vi "Handle Picture Shortcut Activation.vi"(8 "MenuRef":refnum<k9>, 9 "Container State":T1, 10 "state in":T2={"Draw Options"={"Background Color"=16777215, "Grid Color"=13816530, "Angle Units"=enum."Radians", "Draw Solid Background"=TRUE, "Draw Grid"=TRUE, "Grid Spacing"=1.0, "AutoScale"=TRUE, "Fit to Radius"=1.0, "data row options"=[]}}, 11 "data in":T6) -> ()   [LabVIEW 2017, in "NI_Robotics_2D Rangefinder.xctl"]
uses:
  <vilib>/robotics/Controls/2D Rangefinder/NI_Robotics_2D Rangefinder.xctl
  <vilib>/robotics/Controls/2D Rangefinder/_2D Rangefinder Support Files/Data.ctl
  <vilib>/robotics/Controls/2D Rangefinder/_2D Rangefinder Support Files/State.ctl
  <vilib>/robotics/Controls/2D Rangefinder/2D Rangefinder Picture/Draw Options.ctl
  <vilib>/robotics/Controls/Utilities/Angle Units.ctl
  <vilib>/robotics/Controls/2D Rangefinder/2D Rangefinder Picture/Data Row Options.ctl
  <vilib>/_xctls/Container State.ctl
  <vilib>/robotics/Controls/2D Rangefinder/2D Rangefinder Picture/NI_Robotics_2D Rangefinder Picture.lvlib
  <vilib>/_xctls/XControlSupport.lvlib
  <vilib>/robotics/Controls/Utilities/NI_Robotics_Control Utilities.lvlib
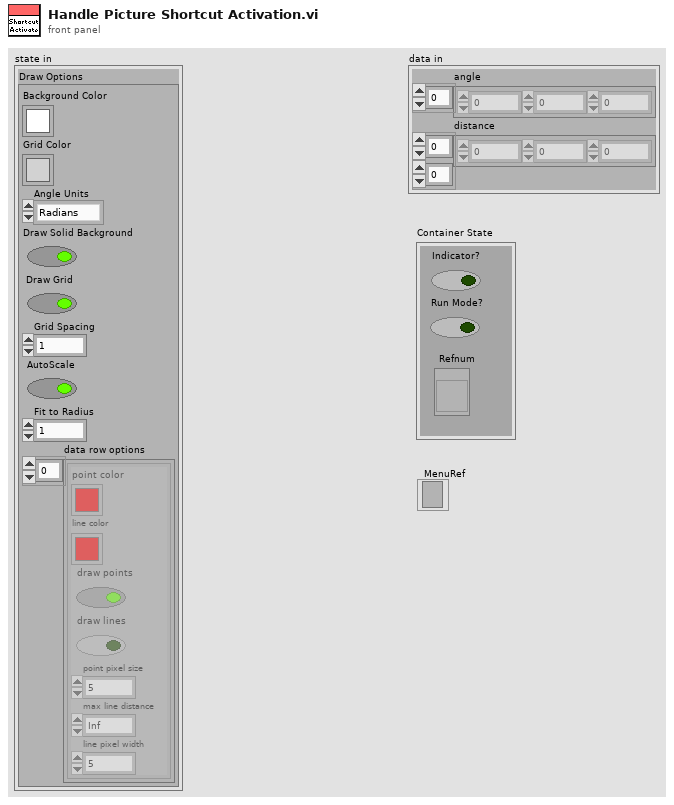
[diagram p1: front panel]
types:
  T1 = typedef "XControlSupport.lvlib/Container State.ctl" = cluster{"Indicator?":bool, "Run Mode?":bool, " Refnum":refnum<vi>}
  T2 = typedef "NI_Robotics_2D Rangefinder.xctl/State.ctl" = cluster{"Draw Options":T3}
  T3 = typedef "NI_Robotics_2D Rangefinder Picture.lvlib/Draw Options.ctl" = cluster{"Background Color":u32, "Grid Color":u32, "Angle Units":T4, "Draw Solid Background":bool, "Draw Grid":bool, "Grid Spacing":dbl, "AutoScale":bool, "Fit to Radius":dbl, "data row options":T5[]}
  T4 = typedef "NI_Robotics_Control Utilities.lvlib/Angle Units.ctl" = enum16{"Radians", "Degrees"}
  T5 = typedef "NI_Robotics_2D Rangefinder Picture.lvlib/Data Row Options.ctl" = cluster{"point color":u32, "line color":u32, "draw points":bool, "draw lines":bool, "point pixel size":u16, "max line distance":dbl, "line pixel width":u16}
  T6 = typedef "NI_Robotics_2D Rangefinder.xctl/Data.ctl" = cluster{"angle":dbl[], "distance":dbl[][]}
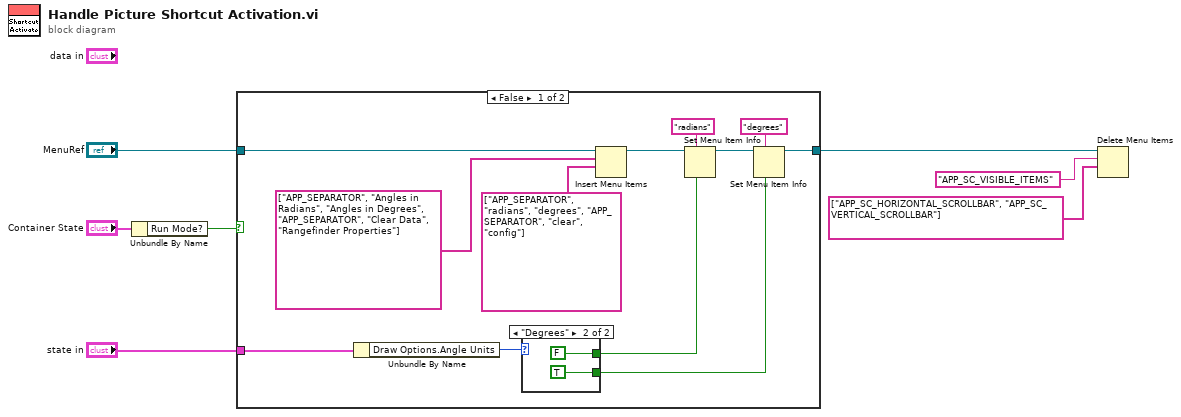
[diagram p0: block diagram]
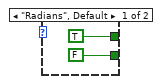
[diagram p2: hidden frame]
diagram:
  n1 = Unbundle By Name("Container State") -> ("Run Mode?"=w2:bool)
  n2 = case shown="False" w2 {
    tunnel: "MenuRef" -> [w19 w24]
    tunnel: [w14 w24] -> w5
    tunnel: "state in" -> [w11 _]
    frame False {
      n3 = Unbundle By Name(w11) -> ("Draw Options.Angle Units"=w10:T4)
      n4 = case shown="\"Degrees\"" w10 {
        tunnel: [TRUE FALSE] -> w9
        tunnel: [FALSE TRUE] -> w8
        frame "Radians", Default {
        }
        frame "Degrees" {
        }
      }
      n5 = Insert Menu Items(7:string[] ["APP_SEPARATOR", "radians", "degrees", "APP_SEPARATOR", "clear", "config"], 8:string[] ["APP_SEPARATOR", "Angles in Radians", "Angles in Degrees", "APP_SEPARATOR", "Clear Data", "Rangefinder Properties"], 9:w19) -> (3:w15:refnum<k9>)  [unwired: 3 in, 2 out]
      n6 = Set Menu Item Info(6:w9, 7:"radians" ("item tag"), 11:w15) -> (3:w16:refnum<k9>)  [unwired: 4 in, 1 out]
      n7 = Set Menu Item Info(6:w8, 7:"degrees" ("item tag"), 11:w16) -> (3:w14:refnum<k9>)  [unwired: 4 in, 1 out]
    }
    frame True {
    }
  }
  n8 = Delete Menu Items(7:string[] ["APP_SC_HORIZONTAL_SCROLLBAR", "APP_SC_VERTICAL_SCROLLBAR"], 8:"APP_SC_VISIBLE_ITEMS", 9:w5) -> ()  [unwired: 1 in, 2 out]
